vi "FTW-Endpoint-Multipart-Ask.vi"(0 "FTW TCP Endpoint":refnum<class "FTW-Endpoint-TCP.lvclass">, 5 "Multipart Message":string[](array[string]), 7 "Read Timeout":i32=100 format="%dmsec", 9 "Write Timeout":i32 format="%dmsec", 11 "error in":errorcluster) -> (4 "FTW Endpoint out":refnum<class "FTW-Endpoint-TCP.lvclass">, 6 "Reply":string[](array[string]), 8 "Read Timed out?":bool, 10 "Write Timed out?":bool, 15 "error out":errorcluster)   [LabVIEW 2013, in "FTW-Endpoint-TCP.lvclass"]
uses:
  FTW-Endpoint-TCP.lvclass
  Ether/FTW-Ether.lvclass
panel:
  # "Inputs"
  # "Outputs"
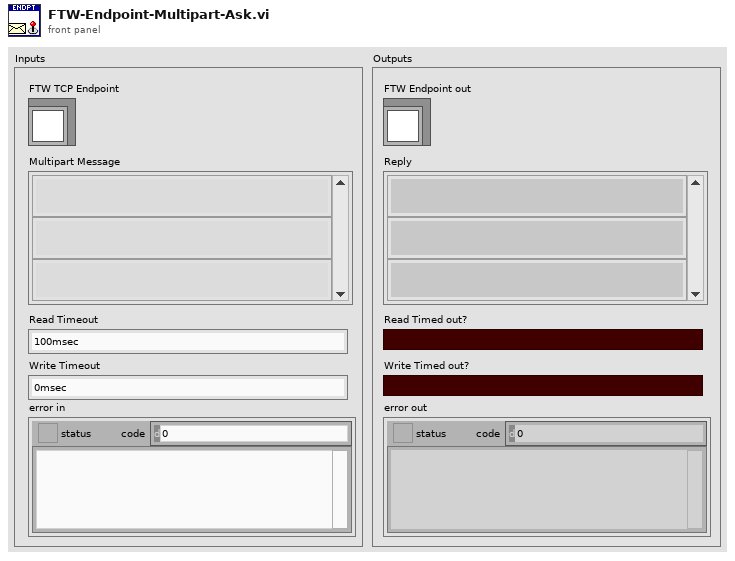
[diagram p1: front panel]
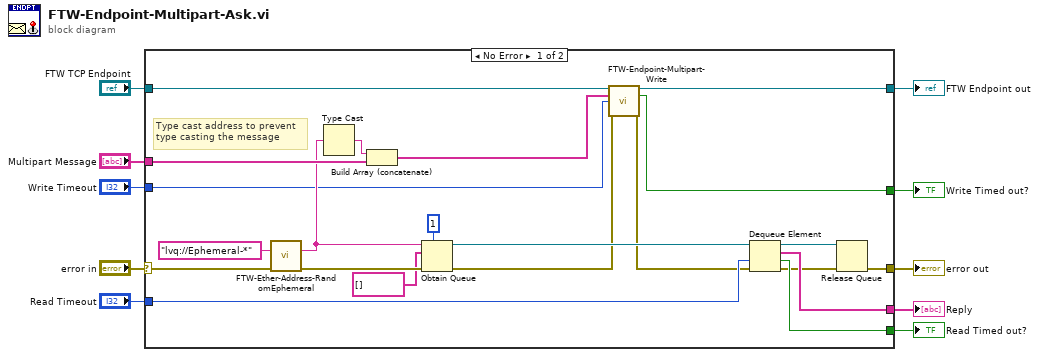
[diagram p0: block diagram]
diagram:
  n1 = case shown="No Error" "error in" {
    selector: "error in" -> [w31 w34]
    tunnel: [w25 w34] -> w10
    tunnel: [w11 w33] -> w8
    tunnel: "FTW TCP Endpoint" -> [w12 w33]
    tunnel: "Multipart Message" -> [w32 _]
    tunnel: "Read Timeout" -> [w30 _]
    tunnel: [w28 _] -> w4
    tunnel: [w29 _] -> w3
    tunnel: [w13 _] -> w2
    tunnel: "Write Timeout" -> [w15 _]
    frame No Error {
      # "Type cast address to prevent\ntype casting the message"
      n2 = call "FTW-Ether-Address-RandomEphemeral.vi"("Endpoint"="lvq://Ephemeral-*" ("Requested Ephemeral Address"), "error in"=w31) -> ("Endpoint with Replacements"=w20:string, "error out"=w23:errorcluster)  [unwired: 12 in]
      n3 = Type Cast(x=w20) -> (*(type *) &x=w22:string)  [unwired: 1 in]
      n4 = Build Array (concatenate)(w22, w32) -> (w17:string[])
      n5 = Obtain Queue(max queue size (-1, unlimited)=1, name (unnamed)=w20, element data type=string[] [], error in (no error)=w23) -> (queue out=w18:refnum<queue>, error out=w16:errorcluster)  [unwired: 1 in, 1 out]
      n6 = call-dynamic "FTW-Endpoint-Multipart-Write.vi"("FTW Endpoint"=w12, "Multipart Message"=w17, "Timeout"=w15, "error in"=w16) -> ("FTW Endpoint out"=w11:refnum<class "FTW-Endpoint-TCP.lvclass">, "Timed out?"=w13:bool, "error out"=w14:errorcluster)  [unwired: 9 in]
      n7 = Dequeue Element(queue=w18, timeout in ms (-1)=w30, error in (no error)=w14) -> (queue out=w27:refnum<queue>, element=w29:string[], timed out?=w28:bool, error out=w26:errorcluster)
      n8 = Release Queue(queue=w27, error in (no error)=w26) -> (error out=w25:errorcluster)  [unwired: 1 in, 2 out]
    }
    frame Error {
    }
  }
  "error out" <- w10
  "FTW Endpoint out" <- w8
  "Read Timed out?" <- w4
  "Reply" <- w3
  "Write Timed out?" <- w2
